vi "CleanLargeFile - LineByLine.vi"() -> ()   [LabVIEW 2019]
uses:
  <vilib>/Utility/file.llb/Read Delimited Spreadsheet (string).vi
  <vilib>/Utility/file.llb/Write Delimited Spreadsheet (string).vi
panel:
  out "Slide":dbl(slide) scale=0.0..1.0
  in  "Target Path":path
  in  "Commit":bool
  in  "Top Header: N Rows":i32
  out "Top Header":string[][](array[string])
  in  "Column Headers":T1(array[cluster])
  out "remaining Header":string[](array[string])
  in  "Path":path
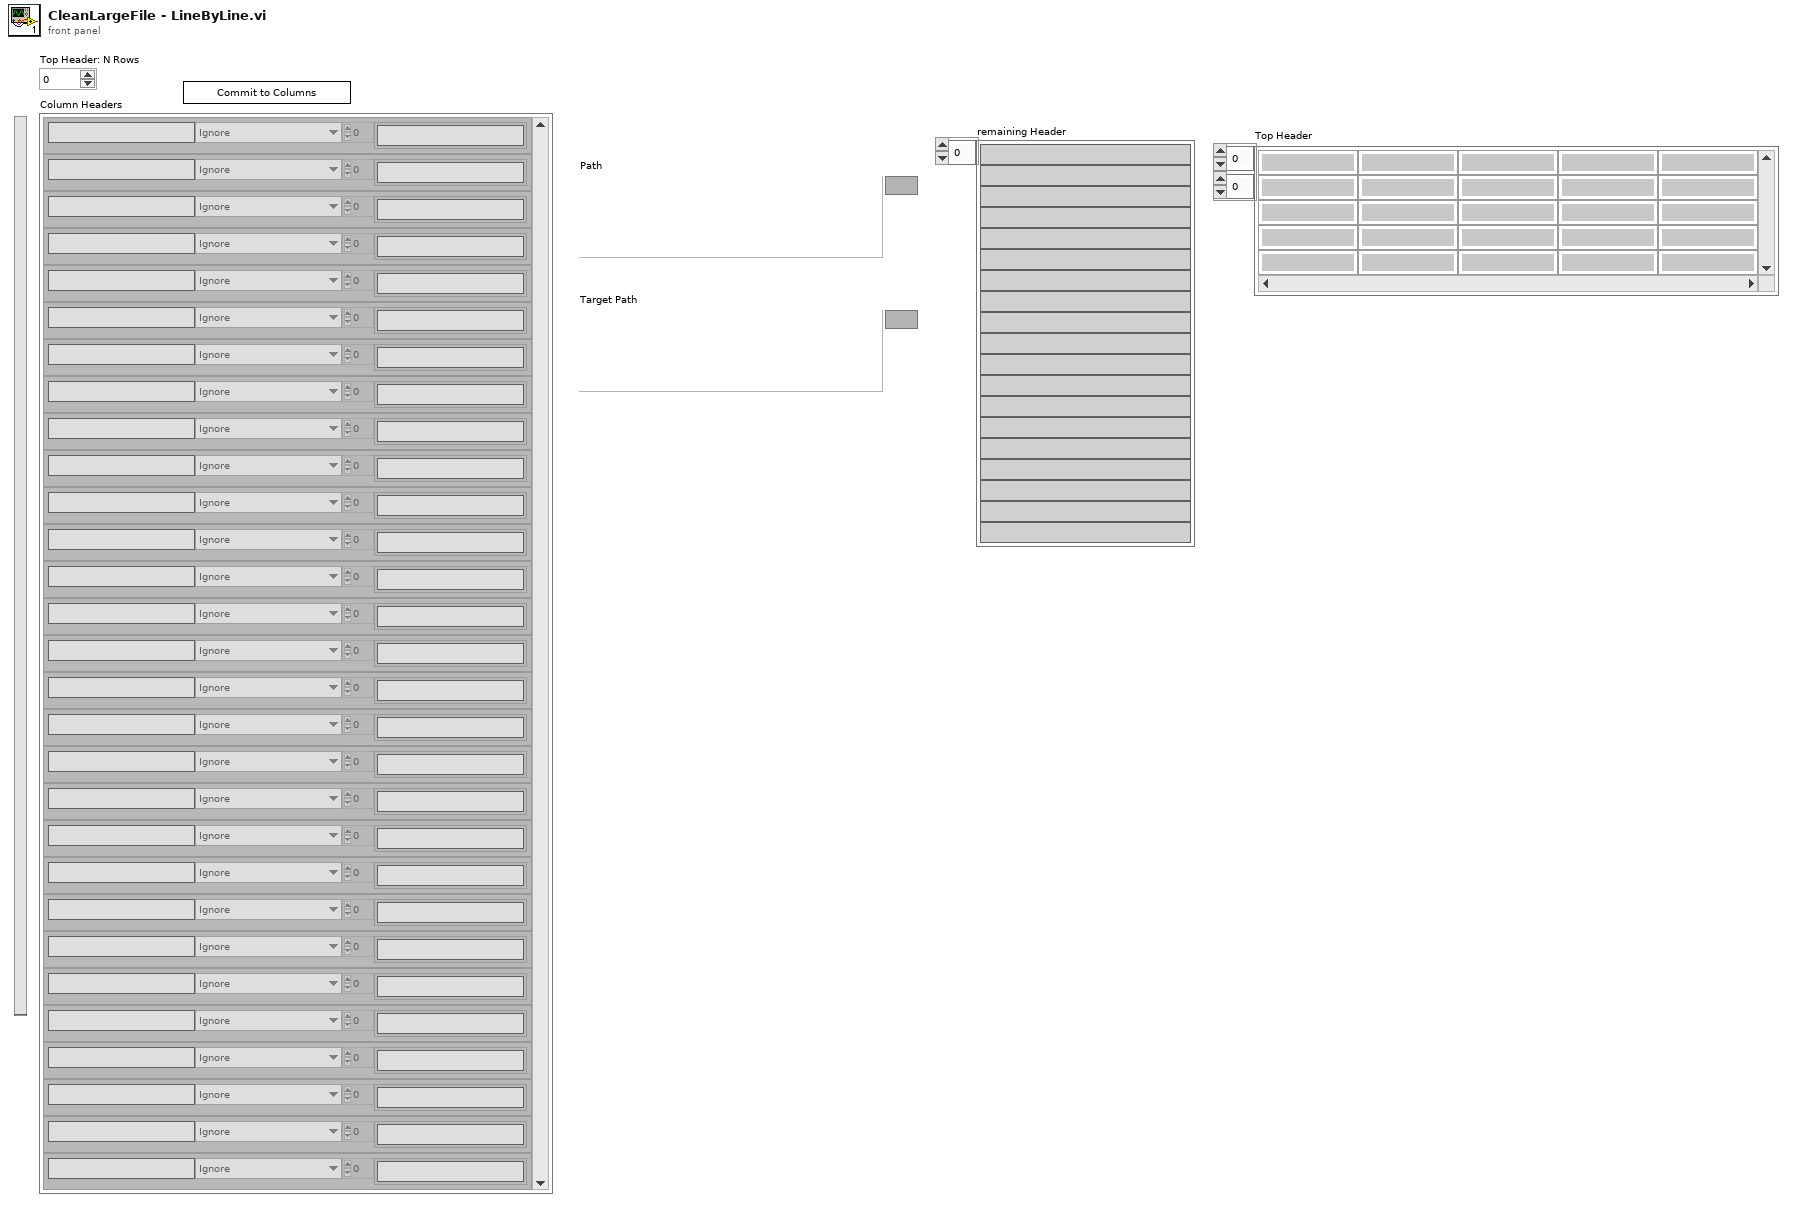
[diagram p1: front panel]
types:
  T1 = cluster{"Column Name":string, "Selector":enum16{"Ignore", "Always Include", "Include Transpose"}, "Unique Elements":string[]}[]
  T2 = cluster{"Column Name":string, "Selector":enum16{"Ignore", "Always Include", "Include Transpose"}, "Unique Elements":string[]}
  T3 = enum16{"Ignore", "Always Include", "Include Transpose"}
  T4 = cluster{"String":string, "Selector":enum16{"Ignore", "Always Include", "Include Transpose"}, string[]}
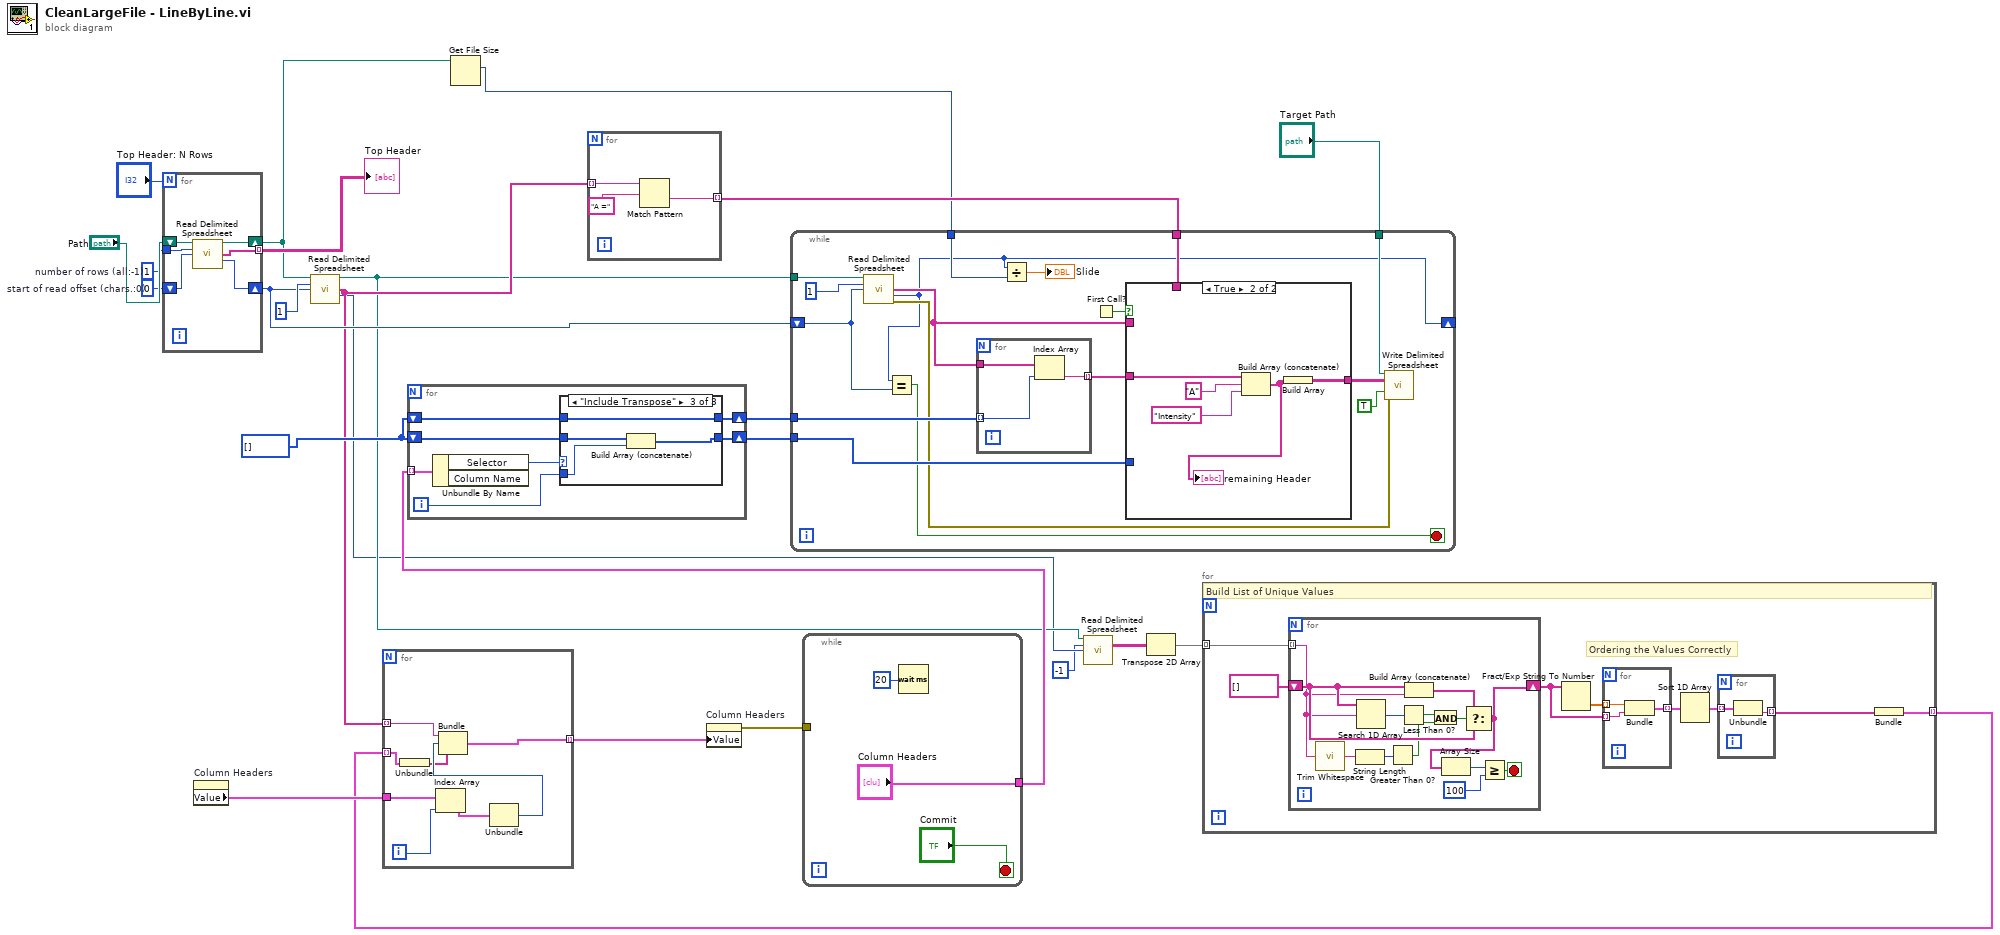
[diagram p0: block diagram]
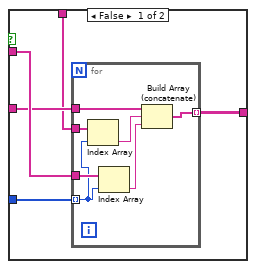
[diagram p2: hidden frame]
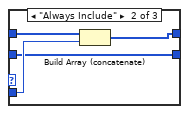
[diagram p4: hidden frame]
diagram:
  w15 = i32[] []
  w23 = 0  # start of read offset (chars.:0)
  w22 = 1  # number of rows (all:-1)
  n1 = for {
    N: "Top Header: N Rows" -> [_]
    tunnel: [w27] -> w24 mode=indexing
    tunnel: w22 -> [w28]
    shift-right: [w29] -> w12
    shift-left: w23 -> [w30]
    shift-right: [w26] -> w8
    shift-left: "Path" -> [w31]
    n2 = call-poly <vilib>:"Read Delimited Spreadsheet.vi"("file path (dialog if empty)"=w31, "number of rows (all:-1)"=w28, "start of read offset (chars.:0)"=w30) -> ("new file path (Not A Path if cancelled)"=w26:path, "first row"=w27:string[], "mark after read (chars.)"=w29:i32)  [unwired: 7 in, 3 out]
  }
  "Top Header" <- w24
  n3 = property on="Column Headers" class="Arr (strict)"() -> ("Value"=w17:T1)  [unwired: 2 in, 2 out]
  n4 = call-poly <vilib>:"Read Delimited Spreadsheet.vi"("file path (dialog if empty)"=w8, "number of rows (all:-1)"=1, "start of read offset (chars.:0)"=w12) -> ("new file path (Not A Path if cancelled)"=w6:path, "first row"=w10:string[], "mark after read (chars.)"=w5:i32)  [unwired: 7 in, 3 out]
  n5 = Get File Size(file=w8) -> (size (in bytes)=w7:i64)  [unwired: 1 in, 2 out]
  n6 = for {
    tunnel: w10 -> [w34] mode=indexing
    tunnel: [w32] -> w9 mode=indexing
    n7 = Match Pattern(string=w34, regular expression="A =") -> (after substring=w32:string)  [unwired: 1 in, 3 out]
  }
  n8 = call-poly <vilib>:"Read Delimited Spreadsheet.vi"("file path (dialog if empty)"=w6, "number of rows (all:-1)"=-1, "start of read offset (chars.:0)"=w5) -> ("all rows"=w3:string[][])  [unwired: 7 in, 5 out]
  n9 = Transpose 2D Array(2D array=w3) -> (transposed array=w2:string[][])
  n10 = for {
    tunnel: w2 -> [w42] mode=indexing
    tunnel: [w40] -> w1 mode=indexing
    # "Ordering the Values Correctly"
    # "Build List of Unique Values"
    n11 = for {
      tunnel: w42 -> [w49] mode=indexing
      shift-right: [w56] -> w36
      shift-left: string[] [] -> [w60]
      stop <- w53 stop-if-true
      n12 = call <vilib>:"Trim Whitespace.vi"("string"=w49) -> ("trimmed string"=w48:string)  [unwired: 1 in]
      n13 = String Length(string=w48) -> (length=w52:i32)
      n14 = Search 1D Array(1D array=w60, element=w49) -> (index of element=w58:i32)  [unwired: 1 in]
      n15 = Greater Than 0?(x=w52) -> (x > 0?=w50:bool)
      n16 = Less Than 0?(x=w58) -> (x < 0?=w57:bool)
      n17 = Build Array (concatenate)(w60, w49) -> (w59:string[])
      n18 = And(x=w57, y=w50) -> (x .and. y?=w51:bool)
      n19 = Select(t=w59, s=w51, f=w60) -> (s? t:f=w56:string[])
      n20 = Array Size(array=w56) -> (size(s)=w55:i32)
      n21 = Greater Or Equal?(x=w55, y=100) -> (x >= y?=w53:bool)
    }
    n22 = Fract/Exp String To Number(string=w36) -> (number=w39:dbl[])  [unwired: 3 in, 1 out]
    n23 = for {
      tunnel: w39 -> [w47] mode=indexing
      tunnel: w36 -> [w46] mode=indexing
      tunnel: [w45] -> w38 mode=indexing
      n24 = Bundle(w47, w46) -> (w45:cluster{dbl, string})  [unwired: 1 in]
    }
    n25 = Sort 1D Array(array=w38) -> (sorted array=w37:cluster{dbl, string}[])
    n26 = for {
      tunnel: w37 -> [w44] mode=indexing
      tunnel: [w43] -> w35 mode=indexing
      n27 = Unbundle(w44) -> (w43:string)  [unwired: 1 out]
    }
    n28 = Bundle(w35) -> (w40:cluster{string[]})  [unwired: 1 in]
  }
  n29 = for {
    tunnel: w10 -> [w68] mode=indexing
    tunnel: [w67] -> w19 mode=indexing
    tunnel: w17 -> [w66]
    tunnel: w1 -> [w62] mode=indexing
    i -> [w65]
    n30 = Unbundle(w62) -> (w61:string[])
    n31 = Index Array(array=w66, index=w65) -> (element=w64:T2)
    n32 = Unbundle(w64) -> ("Selector"=w63:T3)  [unwired: 2 out]
    n33 = Bundle("String"=w68, "Selector"=w63, w61) -> (w67:T4)  [unwired: 1 in]
  }
  n34 = property on="Column Headers" class="Arr (strict)"("Value"=w19) -> (error out=w18:errorcluster)  [unwired: 2 in, 1 out]
  n35 = while {
    tunnel: w18 -> [_]
    tunnel: ["Column Headers"] -> w16
    stop <- "Commit" stop-if-true
    n36 = Wait (ms)(milliseconds to wait=u32 20) -> ()  [unwired: 1 out]
  }
  n37 = for {
    tunnel: w16 -> [w78] mode=indexing
    shift-right: [w75] -> w14
    shift-left: w15 -> [w74]
    shift-right: [w73] -> w13
    shift-left: w15 -> [w72]
    i -> [w76]
    n38 = Unbundle By Name(w78) -> ("Selector"=w77:T3)  [unwired: 1 out]
    n39 = case shown="\"Include Transpose\"" w77 {
      tunnel: w76 -> [_ w84 w88]
      tunnel: [w79 w83 w85] -> w75
      tunnel: w74 -> [w79 w82 w85]
      tunnel: [w80 w81 w87] -> w73
      tunnel: w72 -> [w80 w81 w86]
      frame "Ignore", Default {
      }
      frame "Always Include" {
        n40 = Build Array (concatenate)(w82, w84) -> (w83:i32[])
      }
      frame "Include Transpose" {
        n41 = Build Array (concatenate)(w86, w88) -> (w87:i32[])
      }
    }
  }
  n42 = while {
    tunnel: w6 -> [w105]
    tunnel: w14 -> [w104]
    tunnel: w13 -> [w100]
    shift-right: [w91] -> _
    shift-left: w12 -> [w90]
    tunnel: "Target Path" -> [w96]
    tunnel: w9 -> [w94]
    tunnel: w7 -> [w93]
    stop <- w89 stop-if-true
    n43 = call-poly <vilib>:"Read Delimited Spreadsheet.vi"("file path (dialog if empty)"=w105, "number of rows (all:-1)"=1, "start of read offset (chars.:0)"=w90) -> ("first row"=w99:string[], "mark after read (chars.)"=w91:i32, "error out"=w95:errorcluster)  [unwired: 7 in, 3 out]
    n44 = Equal?(x=w91, y=w90) -> (x = y?=w89:bool)
    n45 = for {
      tunnel: w104 -> [w125] mode=indexing
      tunnel: w99 -> [w124]
      tunnel: [w123] -> w102 mode=indexing
      n46 = Index Array(array=w124, index=w125) -> (element=w123:string)
    }
    n47 = Divide(x=w91, y=w93) -> (x/y=→"Slide":dbl)
    n48 = First Call?() -> (First Call?: T/F=w101:bool)
    n49 = case shown="True" w101 {
      tunnel: w102 -> [w108 w122]
      tunnel: [w107 w120] -> w97
      tunnel: w100 -> [w110 _]
      tunnel: w99 -> [w109 _]
      tunnel: w94 -> [w106 _]
      frame False {
        n50 = for {
          tunnel: w110 -> [w112] mode=indexing
          tunnel: w109 -> [w117]
          tunnel: w108 -> [w114]
          tunnel: [w116] -> w107 mode=indexing
          tunnel: w106 -> [w113]
          n51 = Index Array(array=w113, index=w112) -> (element=w111:string)
          n52 = Index Array(array=w117, index=w112) -> (element=w115:string)
          n53 = Build Array (concatenate)(w114, w111, w115) -> (w116:string[])
        }
      }
      frame True {
        n54 = Build Array (concatenate)(w122, "A" ("regular expression"), "Intensity" ("regular expression")) -> (w119:string[])
        "remaining Header" <- w119
        n55 = Build Array(w119) -> (w120:string[][])
      }
    }
    n56 = call-poly <vilib>:"Write Delimited Spreadsheet.vi"("file path (dialog if empty)"=w96, "2D data"=w97, "append to file? (new file:F)"=TRUE, "error in (no error)"=w95) -> ()  [unwired: 10 in, 2 out]
  }
